vi "Configure IQ vs Slot Measurement Trigger.vi"(0 "VISA resource name":refnum<visa-resource-name>, 1 "Threshold (-30.0)":dbl=-30.0, 2 "Trigger Timeout (0.5)":dbl=0.5, 5 "Instance (1)":i32=1 format="%.0g", 7 "Source (\"IF Power\")":string="IF Power", 9 "Slope (Rising)":i32(ring) items=["Rising", "Falling"], 11 "error in (no error)":errorcluster, 12 "Offset (0.1E-3)":dbl=0.0001, 13 "Gap (0.0)":dbl) -> (4 "VISA resource name out":refnum<visa-resource-name>, 15 "error out":errorcluster)   [LabVIEW 2020, in "Rohde&Schwarz CMXP GPRF.lvlib"]
doc: "Defines the trigger parameters.\n\nAttributes:\nRSCMXPGPRF_ATTR_IQ_VS_SLOT_MEASUREMENT_TRIGGER_SOURCE\nRSCMXPGPRF_ATTR_IQ_VS_SLOT_MEASUREMENT_TRIGGER_SLOPE\nRSCMXPGPRF_ATTR_IQ_VS_SLOT_MEASUREMENT_TRIGGER_THRESHOLD\nRSCMXPGPRF_ATTR_IQ_VS_SLOT_MEASUREMENT_TRIGGER_OFFSET\nRSCMXPGPRF_ATTR_IQ_VS_SLOT_MEASUREMENT_TRIGGER_TIMEOUT\nRSCMXPGPRF_ATTR_IQ_VS_SLOT_MEASUREMENT_TRIGGER_GAP\n\nRemote-control commands:\nTRIGger:GPRF:MEAS<i>:IQVSlot:SOURce\nTRIGger:GPRF:MEAS<i>:IQVSlot:SLOPe\nTRIGger:GPRF:MEAS<i>:IQVSlot:THReshold\nTRIGger:GPRF:MEAS<i>:IQVSlot:OFFSet\nTRIGger:GPRF:MEAS<i>:IQVSlot:TOUT\nTRIGger:GPRF:MEAS<i>:IQVSlot:MGAP"
uses:
  <instrlib>/Rohde&Schwarz CMXP GPRF/Rohde&Schwarz CMXP GPRF.lvlib
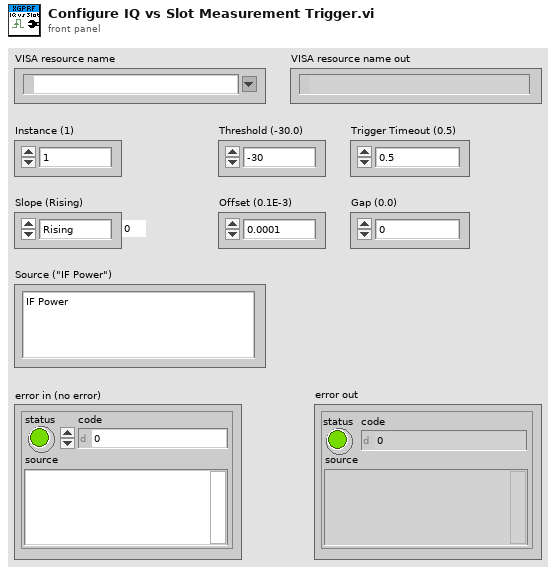
[diagram p1: front panel]
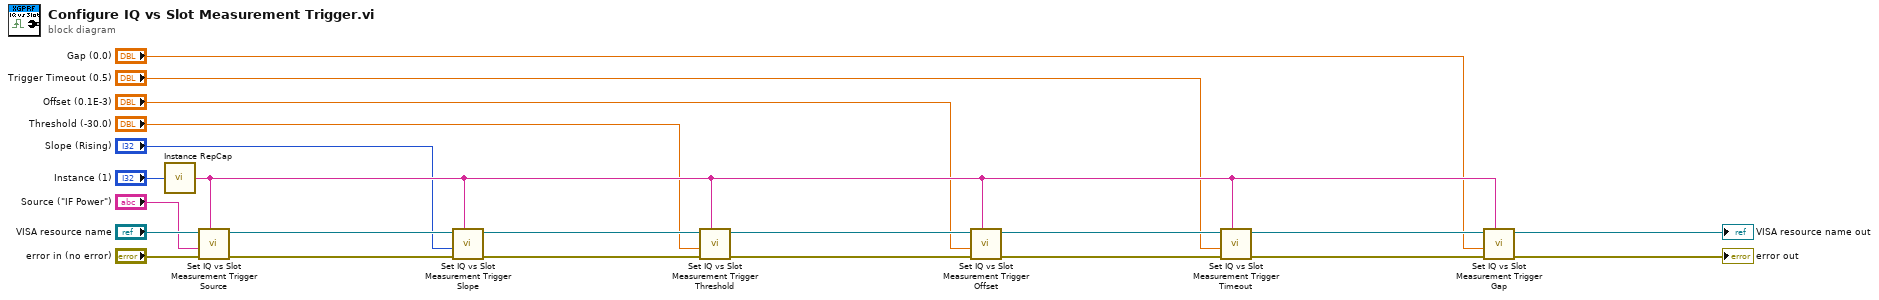
[diagram p0: block diagram]
diagram:
  n1 = call <instrlib>:"Instance RepCap.vi"("Instance in"="Instance (1)") -> ("Instance out"=w22:string)
  n2 = call "Set IQ vs Slot Measurement Trigger Source"("Repeated Capabilities"=w22, "error in (no error)"="error in (no error)", "IQ vs Slot Measurement Trigger Source ()"="Source (\"IF Power\")", "instrument handle"="VISA resource name") -> ("error out"=w18:errorcluster, "instrument handle out"=w19:refnum<visa-resource-name>)  [unwired: 6 in]
  n3 = call "Set IQ vs Slot Measurement Trigger Slope"("Repeated Capabilities"=w22, "error in (no error)"=w18, "IQ vs Slot Measurement Trigger Slope (0 - Rising)"="Slope (Rising)", "instrument handle"=w19) -> ("error out"=w16:errorcluster, "instrument handle out"=w15:refnum<visa-resource-name>)  [unwired: 6 in]
  n4 = call "Set IQ vs Slot Measurement Trigger Threshold"("Repeated Capabilities"=w22, "error in (no error)"=w16, "IQ vs Slot Measurement Trigger Threshold (0.0)"="Threshold (-30.0)", "instrument handle"=w15) -> ("error out"=w13:errorcluster, "instrument handle out"=w14:refnum<visa-resource-name>)  [unwired: 6 in]
  n5 = call "Set IQ vs Slot Measurement Trigger Offset"("Repeated Capabilities"=w22, "error in (no error)"=w13, "IQ vs Slot Measurement Trigger Offset (0.0)"="Offset (0.1E-3)", "instrument handle"=w14) -> ("error out"=w12:errorcluster, "instrument handle out"=w17:refnum<visa-resource-name>)  [unwired: 6 in]
  n6 = call "Set IQ vs Slot Measurement Trigger Timeout"("Repeated Capabilities"=w22, "error in (no error)"=w12, "IQ vs Slot Measurement Trigger Timeout (0.0)"="Trigger Timeout (0.5)", "instrument handle"=w17) -> ("error out"=w20:errorcluster, "instrument handle out"=w21:refnum<visa-resource-name>)  [unwired: 6 in]
  n7 = call "Set IQ vs Slot Measurement Trigger Gap"("Repeated Capabilities"=w22, "error in (no error)"=w20, "IQ vs Slot Measurement Trigger Gap (0.0)"="Gap (0.0)", "instrument handle"=w21) -> ("error out"=→"error out":errorcluster, "instrument handle out"=→"VISA resource name out":refnum<visa-resource-name>)  [unwired: 6 in]
